vi "Teleop.vi"(10 "Match Info":T1={"Autonomous Elapsed Seconds"=0.0, "TeleOp Elapsed Seconds"=0.0, "Disabled Elapsed Seconds"=0.0, "Visited Autonomous"=FALSE, "Visited TeleOp"=FALSE, "Visited Disabled"=FALSE, "Autonomous Settings"={"Autonomous Style"=enum."Independent", "VI Refnum"=refnum}}, 11 "Call Context":T2) -> ()   [LabVIEW 2020]
doc: "This VI is called for each TeleOp packet received from the DS where the robot is not disabled. It is often used to read from the joysticks and update I/O or to update setpoints for timed control loops. It should complete and return within 20 milliseconds or it may miss DS packets."
uses:
  <vilib>/Rock Robotics/WPI/DriverStation/WPI_DriverStationDerivedRobotMode.ctl
  <vilib>/Rock Robotics/WPI/DriverStation/WPI_DriverStationMatch Info.ctl
  <vilib>/Rock Robotics/Network Tables/NT Read Boolean.vi
  <vilib>/Rock Robotics/Network Tables/NT Read Number.vi
  <vilib>/Rock Robotics/WPI/Utilities/WPI_GetSetVariantRefNum.vi
  <vilib>/Rock Robotics/Network Tables/NT Write Boolean Array.vi
  <vilib>/Rock Robotics/Network Tables/NT Write Numeric Array.vi
panel:
  in  "Gear Ratio":dbl=740.0 format="%#_13g"
  in  "Wheelbase":dbl=17.25
  in  "Trackwidth":dbl=19.5
  in  "upper limit":dbl=0.02
  in  "lower limit":dbl=-0.02
  out "Angle Back Left":dbl
  out "Angle Back Right":dbl
  out "Angle Front Right":dbl
  out "Angle Front Left":dbl
  out "Speed Back Left":dbl
  out "Speed Back Right":dbl
  out "Speed Front Right":dbl
  out "Speed Front Left":dbl
  in  "reverse steer":bool
  in  "reverse encoder":bool
  in  "ScaleSpeed":dbl=1.0
  out "Sample Slider 0":dbl(slide) scale=0.0..5.0
  out "Sample Boolean 1":bool
  out "Sample Boolean 0":bool
  # "740 guess"
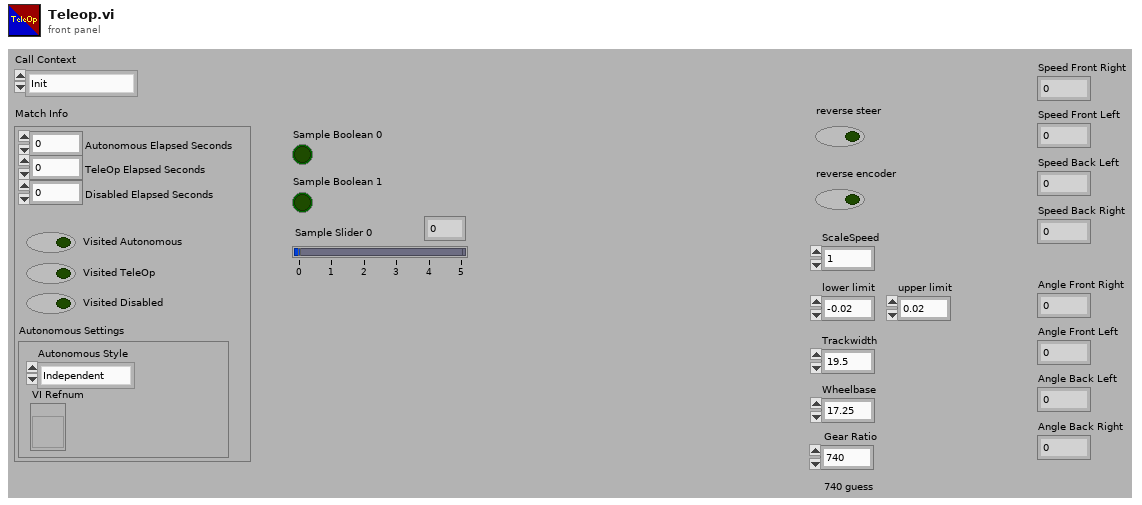
[diagram p1: front panel]
types:
  T1 = typedef "WPI_DriverStationMatch Info.ctl" = cluster{"Autonomous Elapsed Seconds":dbl, "TeleOp Elapsed Seconds":dbl, "Disabled Elapsed Seconds":dbl, "Visited Autonomous":bool, "Visited TeleOp":bool, "Visited Disabled":bool, "Autonomous Settings":cluster{"Autonomous Style":enum16{"Iterative", "Independent"}, "VI Refnum":refnum<vi>}}
  T2 = typedef "WPI_DriverStationDerivedRobotMode.ctl" = enum16{"Init", "Execute", "Stop"}
  T3 = typedef "WPI_JoystickDevRef.ctl" = cluster{"Device":T4}
  T4 = typedef "WPI_JoystickDeviceEnum.ctl" = enum16{"USB 0", "USB 1", "USB 2", "USB 3", "USB 4", "USB 5"}
  T5 = typedef "WPI_MotorControlDeviceRef.ctl" = cluster{"DeviceStatus":errorcluster, "Type":T6, "PWM":cluster{"PWM Channel":T7, "DeadBand":T8}, "CAN":cluster{"Device Number":u8, "SetOutput VI Ref":variant, "GetOutput VI Ref":variant, "Enable VI Ref":variant, "Disable VI Ref":variant, "Data":variant}, "Invert":bool, "DIO PWM":cluster{"PWM \"Enable\" Channel":T7, "DIOChannel":T9, "PWM Rate":dbl}}
  T6 = typedef "WPI_MotorControlType.ctl" = enum16{"PWM", "CAN", "DIO PWM"}
  T7 = typedef "FPGA_DIOPWMChannel.ctl" = enum8{"PWM 0", "PWM 1", "PWM 2", "PWM 3", "PWM 4", "PWM 5", "PWM 6", "PWM 7", "PWM 8", "PWM 9", "PWM MXP 0", "PWM MXP 1", "PWM MXP 2", "PWM MXP 3", "PWM MXP 4", "PWM MXP 5", "PWM MXP 6", "PWM MXP 7", "PWM MXP 8", "PWM MXP 9", "Invalid"}
  T8 = typedef "WPI_PWMDeadband.ctl" = cluster{"Name":string, "maxPositivePwm":i32, "minPositivePwm":i32, "centerPwm":i32, "maxNegativePwm":i32, "minNegativePwm":i32, "angularRange":u16}
  T9 = typedef "FPGA_DIOChannel.ctl" = enum8{"DIO 0", "DIO 1", "DIO 2", "DIO 3", "DIO 4", "DIO 5", "DIO 6", "DIO 7", "DIO 8", "DIO 9", "DIO MXP 0", "DIO MXP 1", "DIO MXP 2", "DIO MXP 3", "DIO MXP 4", "DIO MXP 5", "DIO MXP 6", "DIO MXP 7", "DIO MXP 8", "DIO MXP 9", "DIO MXP 10", "DIO MXP 11", "DIO MXP 12", "DIO MXP 13", "DIO MXP 14", "DIO MXP 15", "SPI Port CS1", "SPI Port CS2", "SPI Port CS3", "SPI Port MISO", "SPI Port MOSI", "Invalid"}
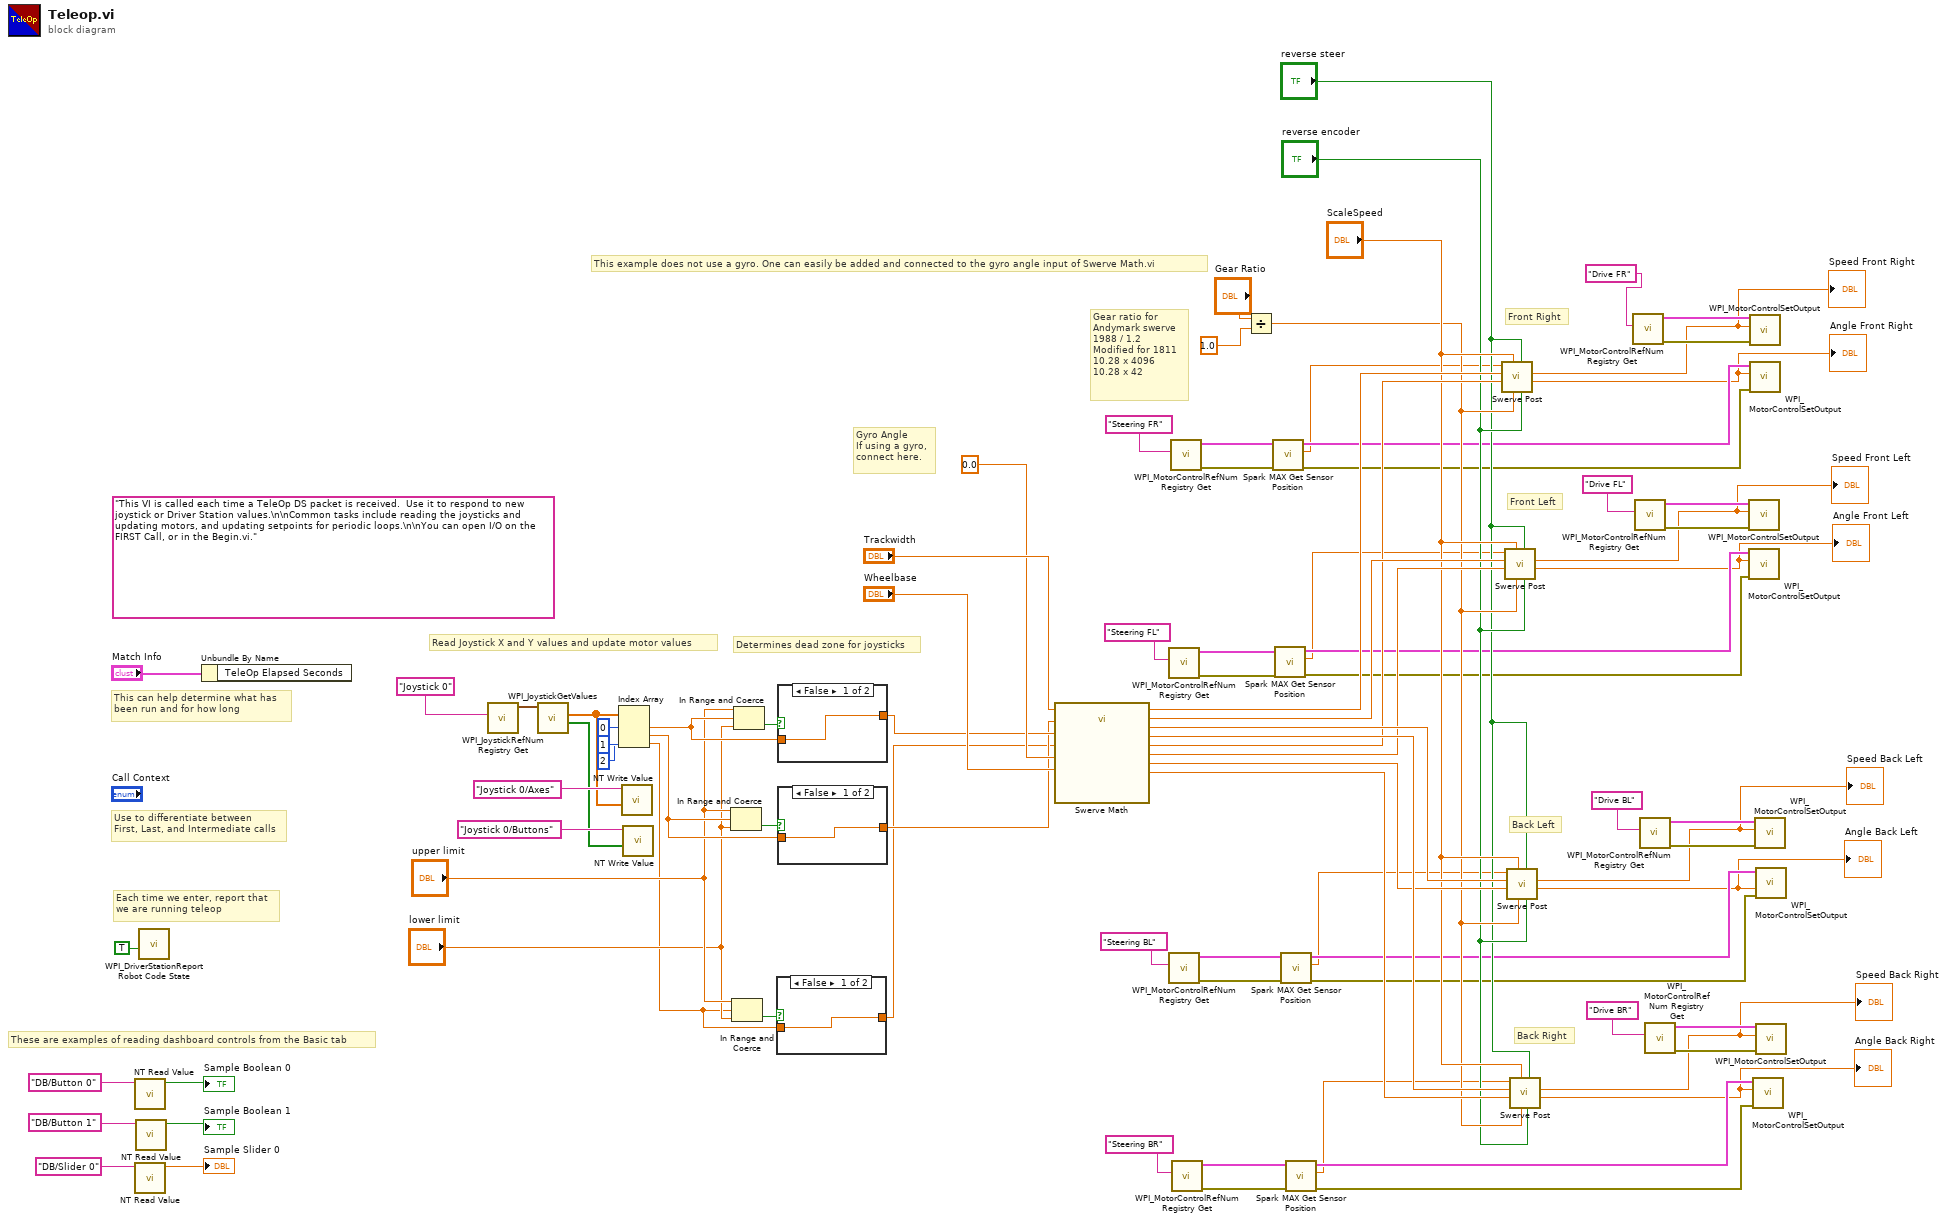
[diagram p0: block diagram]
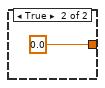
[diagram p2: hidden frame]
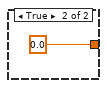
[diagram p3: hidden frame]
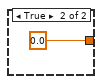
[diagram p4: hidden frame]
diagram:
  (unwired) "This VI is called each time a TeleOp DS packet is received.  Use it to respond to new joystick or Driver Station values.\n\nCommon tasks include reading the joysticks and updating motors, and updating setpoints for periodic loops.\n\nYou can open I/O on the FIRST Call, or in the Begin.vi."
  # "Gyro Angle\nIf using a gyro,\nconnect here."
  # "Determines dead zone for joysticks"
  # "Read Joystick X and Y values and update motor values"
  # "Gear ratio for\nAndymark swerve\n1988 / 1.2\nModified for 1811\n10.28 x 4096\n10.28 x 42"
  # "Back Right"
  # "Back Left"
  # "Front Left"
  # "Front Right"
  # "This example does not use a gyro. One can easily be added and connected to the gyro angle input of Swerve Math.vi"
  # "These are examples of reading dashboard controls from the Basic tab"
  # "Each time we enter, report that\nwe are running teleop"
  # "Use to differentiate between\nFirst, Last, and Intermediate calls"
  # "This can help determine what has\nbeen run and for how long"
  n1 = call-poly <vilib>:"NT Read Value.vi"("name"="DB/Button 0" ("refnum name")) -> ("value"=→"Sample Boolean 0":bool)  [unwired: 8 in, 2 out]
  n2 = call-poly <vilib>:"NT Read Value.vi"("name"="DB/Slider 0" ("refnum name")) -> ("value"=→"Sample Slider 0":dbl)  [unwired: 8 in, 2 out]
  n3 = call-poly <vilib>:"NT Read Value.vi"("name"="DB/Button 1" ("refnum name")) -> ("value"=→"Sample Boolean 1":bool)  [unwired: 8 in, 2 out]
  n4 = call <vilib>:"WPI_DriverStationReport Robot Code State.vi"("TeleOp"=TRUE ("Autonomous")) -> ()  [unwired: 10 in, 1 out]
  n5 = Unbundle By Name("Match Info") -> ()  [unwired: 1 out]
  n6 = call <vilib>:"WPI_JoystickRefNum Registry Get.vi"("refnum name"="Joystick 0") -> ("JoystickDevRef"=w26:T3)  [unwired: 1 in, 9 out]
  n7 = call <vilib>:"WPI_JoystickGetValues.vi"("JoystickDevRef"=w26) -> ("Buttons"=w22:bool[], "Axes"=w23:dbl[])  [unwired: 6 in, 3 out]
  n8 = Index Array(array=w23, index #1=0 ("index"), index #2=1 ("index"), index #3=2 ("index")) -> (element #1=w17:dbl, element #2=w18:dbl, element #3=w14:dbl)
  n9 = call-poly <vilib>:"NT Write Value.vi"("value"=w23, "name"="Joystick 0/Axes" ("Name")) -> ()  [unwired: 9 in, 1 out]
  n10 = call-poly <vilib>:"NT Write Value.vi"("value"=w22, "name"="Joystick 0/Buttons" ("Name")) -> ()  [unwired: 9 in, 1 out]
  n11 = In Range and Coerce(upper limit="upper limit", x=w18, lower limit="lower limit") -> (In Range?=w20:bool)  [unwired: 1 out]
  n12 = In Range and Coerce(upper limit="upper limit", x=w14, lower limit="lower limit") -> (In Range?=w21:bool)  [unwired: 1 out]
  n13 = In Range and Coerce(upper limit="upper limit", x=w17, lower limit="lower limit") -> (In Range?=w19:bool)  [unwired: 1 out]
  n14 = case shown="False" w21 {
    tunnel: [w90 0.0 ("Gyro Angle")] -> w1
    tunnel: w14 -> [w90 _]
    frame False {
    }
    frame True {
    }
  }
  n15 = case shown="False" w19 {
    tunnel: [w92 0.0 ("Gyro Angle")] -> w3
    tunnel: w17 -> [w92 _]
    frame False {
    }
    frame True {
    }
  }
  n16 = case shown="False" w20 {
    tunnel: [w94 0.0 ("Gyro Angle")] -> w2
    tunnel: w18 -> [w94 _]
    frame False {
    }
    frame True {
    }
  }
  n17 = call "Swerve Math.vi"("Trackwidth (W)"="Trackwidth", "Wheelbase (L)"="Wheelbase", "Y -FWD"=w2, "X1 STR"=w3, "X2 RCW"=w1, "Gyro Angle in degrees"=0.0 ("Gyro Angle")) -> ("wa3"=w71:dbl, "wa4"=w70:dbl, "ws1"=w76:dbl, "ws2"=w75:dbl, "ws3"=w74:dbl, "ws4"=w77:dbl, "wa2"=w72:dbl, "wa1"=w73:dbl)  [unwired: 2 in]
  n18 = call <vilib>:"WPI_MotorControlRefNum Registry Get.vi"("refnum name"="Steering FL") -> ("error out"=w46:errorcluster, "MotorControlDevRef"=w47:T5)  [unwired: 9 in]
  n19 = call <vilib>:"WPI_MotorControlRefNum Registry Get.vi"("refnum name"="Steering BL") -> ("error out"=w52:errorcluster, "MotorControlDevRef"=w53:T5)  [unwired: 9 in]
  n20 = call <vilib>:"WPI_MotorControlRefNum Registry Get.vi"("refnum name"="Steering FR") -> ("error out"=w42:errorcluster, "MotorControlDevRef"=w43:T5)  [unwired: 9 in]
  n21 = call <vilib>:"WPI_MotorControlRefNum Registry Get.vi"("refnum name"="Steering BR") -> ("error out"=w54:errorcluster, "MotorControlDevRef"=w55:T5)  [unwired: 9 in]
  n22 = Divide(x="Gear Ratio", y=1.0) -> (x/y=w66:dbl)
  n23 = call <vilib>:"Spark MAX Get Sensor Position.vi"("error in (no error)"=w42, "MotorControlDevRef in"=w43) -> ("error out"=w41:errorcluster, "Sensor Position"=w31:dbl, "MotorControlDevRef out"=w40:T5)  [unwired: 6 in, 1 out]
  n24 = call <vilib>:"Spark MAX Get Sensor Position.vi"("error in (no error)"=w46, "MotorControlDevRef in"=w47) -> ("error out"=w45:errorcluster, "Sensor Position"=w30:dbl, "MotorControlDevRef out"=w44:T5)  [unwired: 6 in, 1 out]
  n25 = call <vilib>:"Spark MAX Get Sensor Position.vi"("error in (no error)"=w52, "MotorControlDevRef in"=w53) -> ("error out"=w51:errorcluster, "Sensor Position"=w29:dbl, "MotorControlDevRef out"=w50:T5)  [unwired: 6 in, 1 out]
  n26 = call <vilib>:"Spark MAX Get Sensor Position.vi"("error in (no error)"=w54, "MotorControlDevRef in"=w55) -> ("error out"=w49:errorcluster, "Sensor Position"=w28:dbl, "MotorControlDevRef out"=w48:T5)  [unwired: 6 in, 1 out]
  n27 = call "Swerve Post.vi"("reverse encoder"="reverse encoder", "reverse steer"="reverse steer", "gear ratio"=w66, "ScaleSpeed"="ScaleSpeed", "wa in"=w73, "ws in"=w76, "encoder in"=w31) -> ("wa out"=w33:dbl, "ws out 0-1"=w32:dbl)  [unwired: 3 in]
  "Speed Front Right" <- w32
  "Angle Front Right" <- w33
  n28 = call "Swerve Post.vi"("reverse encoder"="reverse encoder", "reverse steer"="reverse steer", "gear ratio"=w66, "ScaleSpeed"="ScaleSpeed", "wa in"=w72, "ws in"=w75, "encoder in"=w30) -> ("wa out"=w35:dbl, "ws out 0-1"=w34:dbl)  [unwired: 3 in]
  "Speed Front Left" <- w34
  "Angle Front Left" <- w35
  n29 = call "Swerve Post.vi"("reverse encoder"="reverse encoder", "reverse steer"="reverse steer", "gear ratio"=w66, "ScaleSpeed"="ScaleSpeed", "wa in"=w71, "ws in"=w74, "encoder in"=w29) -> ("wa out"=w37:dbl, "ws out 0-1"=w36:dbl)  [unwired: 3 in]
  "Speed Back Left" <- w36
  "Angle Back Left" <- w37
  n30 = call "Swerve Post.vi"("reverse encoder"="reverse encoder", "reverse steer"="reverse steer", "gear ratio"=w66, "ScaleSpeed"="ScaleSpeed", "wa in"=w70, "ws in"=w77, "encoder in"=w28) -> ("wa out"=w39:dbl, "ws out 0-1"=w38:dbl)  [unwired: 3 in]
  "Speed Back Right" <- w38
  "Angle Back Right" <- w39
  n31 = call <vilib>:"WPI_MotorControlRefNum Registry Get.vi"("refnum name"="Drive FR") -> ("error out"=w63:errorcluster, "MotorControlDevRef"=w64:T5)  [unwired: 9 in]
  n32 = call <vilib>:"WPI_MotorControlRefNum Registry Get.vi"("refnum name"="Drive FL") -> ("error out"=w61:errorcluster, "MotorControlDevRef"=w62:T5)  [unwired: 9 in]
  n33 = call <vilib>:"WPI_MotorControlRefNum Registry Get.vi"("refnum name"="Drive BL") -> ("error out"=w59:errorcluster, "MotorControlDevRef"=w60:T5)  [unwired: 9 in]
  n34 = call <vilib>:"WPI_MotorControlRefNum Registry Get.vi"("refnum name"="Drive BR") -> ("error out"=w57:errorcluster, "MotorControlDevRef"=w58:T5)  [unwired: 9 in]
  n35 = call <vilib>:"WPI_MotorControlSetOutput.vi"("error in (no error)"=w61, "Output"=w34, "MotorControlDevRef"=w62) -> ()  [unwired: 6 in, 3 out]
  n36 = call <vilib>:"WPI_MotorControlSetOutput.vi"("error in (no error)"=w45, "Output"=w35, "MotorControlDevRef"=w44) -> ()  [unwired: 6 in, 3 out]
  n37 = call <vilib>:"WPI_MotorControlSetOutput.vi"("error in (no error)"=w63, "Output"=w32, "MotorControlDevRef"=w64) -> ()  [unwired: 6 in, 3 out]
  n38 = call <vilib>:"WPI_MotorControlSetOutput.vi"("error in (no error)"=w41, "Output"=w33, "MotorControlDevRef"=w40) -> ()  [unwired: 6 in, 3 out]
  n39 = call <vilib>:"WPI_MotorControlSetOutput.vi"("error in (no error)"=w49, "Output"=w39, "MotorControlDevRef"=w48) -> ()  [unwired: 6 in, 3 out]
  n40 = call <vilib>:"WPI_MotorControlSetOutput.vi"("error in (no error)"=w59, "Output"=w36, "MotorControlDevRef"=w60) -> ()  [unwired: 6 in, 3 out]
  n41 = call <vilib>:"WPI_MotorControlSetOutput.vi"("error in (no error)"=w51, "Output"=w37, "MotorControlDevRef"=w50) -> ()  [unwired: 6 in, 3 out]
  n42 = call <vilib>:"WPI_MotorControlSetOutput.vi"("error in (no error)"=w57, "Output"=w38, "MotorControlDevRef"=w58) -> ()  [unwired: 6 in, 3 out]
